vi "Update display target.vi"(8 "error in (no error)":errorcluster, 11 "StageSPIM in":refnum<class "StageSPIM.lvclass">) -> (0 "error out":errorcluster, 3 "StageSPIM out":refnum<class "StageSPIM.lvclass">)   [LabVIEW 2012, in "StageSPIM.lvclass"]
uses:
  StageSPIM.lvclass
  StageSPIM.lvclass/StageSPIM.ctl
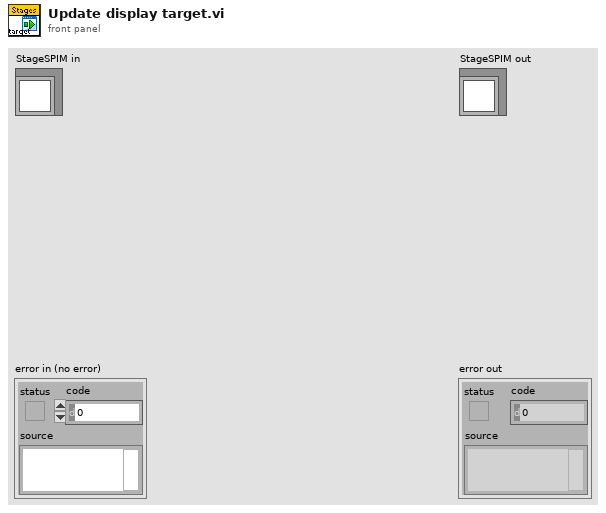
[diagram p1: front panel]
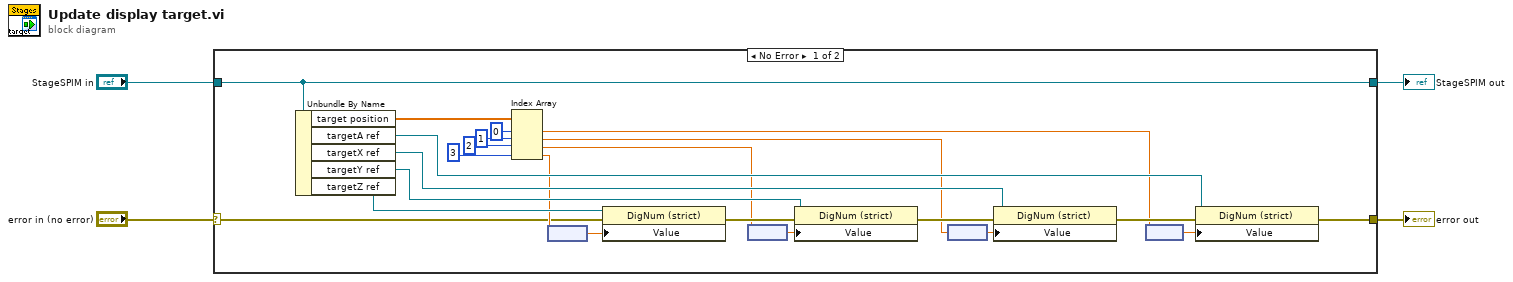
[diagram p0: block diagram]
diagram:
  n1 = case shown="No Error" "error in (no error)" {
    selector: "error in (no error)" -> [w6 w29]
    tunnel: [w5 w29] -> w3
    tunnel: [w7 w28] -> w1
    tunnel: "StageSPIM in" -> [w7 w28]
    frame No Error {
      n2 = Unbundle By Name(w7) -> ("target position"=w27:dbl[], "targetA ref"=w19:refnum<vi>, "targetX ref"=w20:refnum<vi>, "targetY ref"=w21:refnum<vi>, "targetZ ref"=w22:refnum<vi>)
      n3 = Index Array(array=w27, index #1=0 ("index"), index #2=1 ("index"), index #3=2 ("index"), index #4=3 ("index")) -> (element #1=w8:dbl, element #2=w10:dbl, element #3=w12:dbl, element #4=w14:dbl)
      n4 = node(w14) -> (w15:dbl[unit])
      n5 = property class="DigNum (strict)"(reference=w22, error in=w6, "Value"=w15) -> (error out=w18:errorcluster)  [unwired: 1 out]
      n6 = node(w12) -> (w13:dbl[unit])
      n7 = property class="DigNum (strict)"(reference=w21, error in=w18, "Value"=w13) -> (error out=w17:errorcluster)  [unwired: 1 out]
      n8 = node(w10) -> (w11:dbl[unit])
      n9 = property class="DigNum (strict)"(reference=w20, error in=w17, "Value"=w11) -> (error out=w16:errorcluster)  [unwired: 1 out]
      n10 = node(w8) -> (w9:dbl[unit])
      n11 = property class="DigNum (strict)"(reference=w19, error in=w16, "Value"=w9) -> (error out=w5:errorcluster)  [unwired: 1 out]
    }
    frame Error {
    }
  }
  "error out" <- w3
  "StageSPIM out" <- w1
